vi "Close.vi"(8 "error in":errorcluster, 11 "Thermometer DAQmx Config in":refnum<class "Thermometer DAQmx Config.lvclass">) -> (0 "error out":errorcluster, 3 "Thermometer DAQmx Config out":refnum<class "Thermometer DAQmx Config.lvclass">)   [LabVIEW 2023, in "Thermometer.lvlib" / "Thermometer DAQmx.lvlib" / "Thermometer DAQmx Config.lvclass"]
uses:
  Thermometer DAQmx Config.lvclass
  Thermometer DAQmx Config.lvclass/Thermometer DAQmx Config.ctl
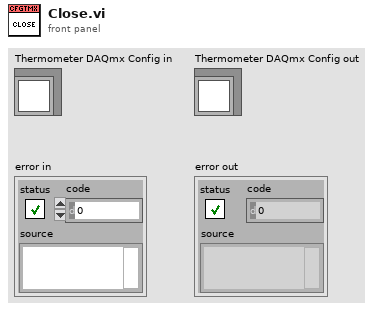
[diagram p1: front panel]
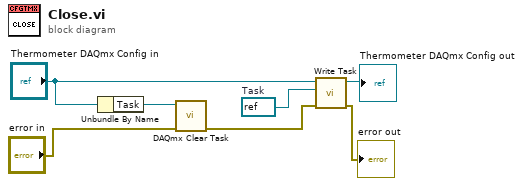
[diagram p0: block diagram]
diagram:
  w4 = refnum<k21> refnum  # Task
  n1 = Unbundle By Name("Thermometer DAQmx Config in") -> ("Task"=w7:refnum<k21>)
  n2 = call <vilib>:"DAQmx Clear Task.vi"("task in"=w7, "error in"="error in") -> ("error out"=w3:errorcluster)  [unwired: 13 in]
  n3 = call "Write Task.vi"("error in (no error)"=w3, "Task"=w4, "Thermometer DAQmx Config in"="Thermometer DAQmx Config in") -> ("error out"=→"error out":errorcluster, "Thermometer DAQmx Config out"=→"Thermometer DAQmx Config out":refnum<class "Thermometer DAQmx Config.lvclass">)  [unwired: 7 in]
